vi "Close Device Core.vi"(8 "error in (no error)":errorcluster, 11 "CS++Scope in":refnum<class "CS++Scope.lvclass">) -> (0 "error out":errorcluster, 3 "CS++Scope out":refnum<class "CS++Scope.lvclass">)   [LabVIEW 2016, in "CS++Scope.lvlib" / "CS++Scope.lvclass"]
doc: "Close device driver connection."
uses:
  CS++Scope.lvclass
  CSPP_Core/Actors/CS++DeviceActor/CS++DeviceActor.lvclass
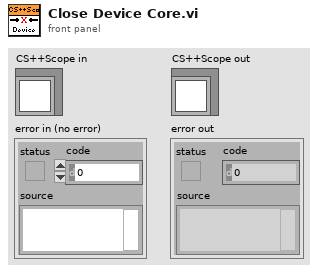
[diagram p1: front panel]
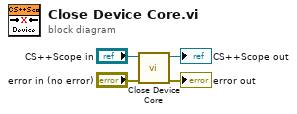
[diagram p0: block diagram]
diagram:
  n1 = call-parent "Close Device Core.vi"("error in (no error)"="error in (no error)", "CS++DeviceActor in"="CS++Scope in") -> ("error out"=→"error out":errorcluster, "CS++DeviceActor out"=→"CS++Scope out":refnum<class "CS++Scope.lvclass">)  [unwired: 8 in]
